vi "Test_Combined_Convert_CameraAngle_to_Flywheel_Velocity.vi"() -> ()   [LabVIEW 2019]
panel:
  in  "angle":dbl
  in  "terminal height":dbl
  out "Test Plot":cluster{dbl[], dbl[]}[](graph)
  out "a2":dbl
  out "d":dbl
  in  "StopValue":dbl=25.0
  in  "StartValue":dbl=-25.0
  in  "h1":dbl=20.56
  in  "h2":dbl=98.25
  in  "a1":dbl
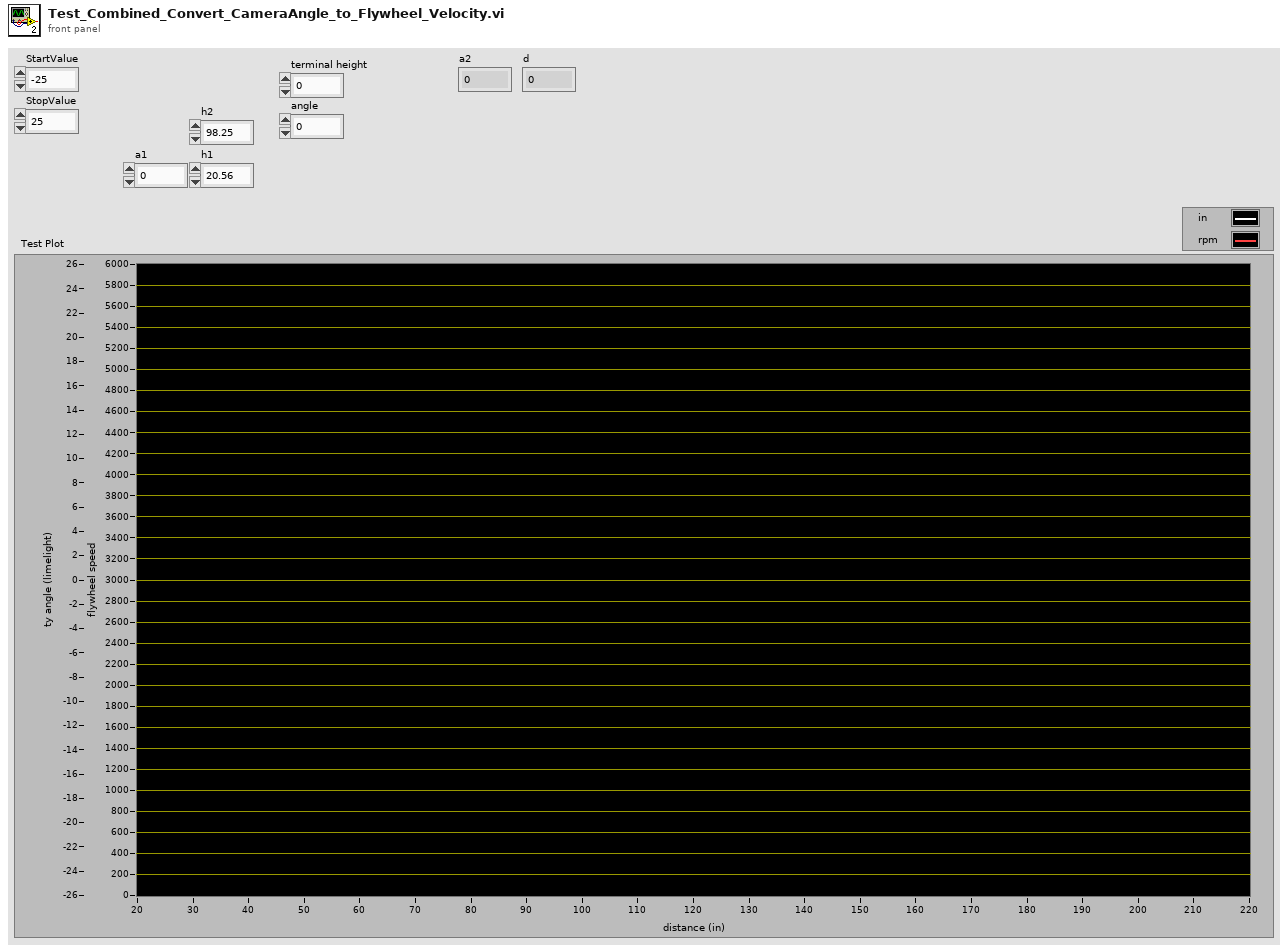
[diagram p1: front panel]
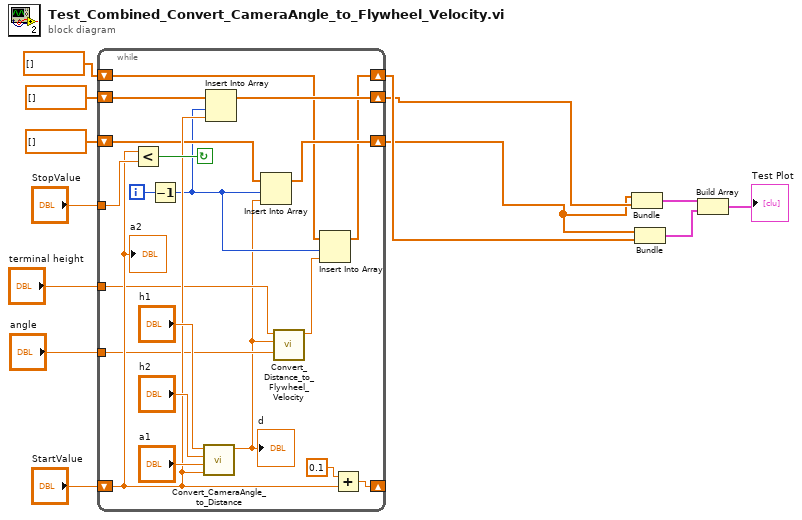
[diagram p0: block diagram]
diagram:
  n1 = while {
    shift-right: [w29] -> _
    shift-left: "StartValue" -> [w25]
    tunnel: "StopValue" -> [w28]
    shift-right: [w22] -> w2
    shift-left: dbl[] [] -> [w24]
    shift-right: [w21] -> w1
    shift-left: dbl[] [] -> [w23]
    shift-right: [w17] -> w3
    shift-left: dbl[] [] -> [w18]
    tunnel: "terminal height" -> [w16]
    tunnel: "angle" -> [w15]
    i -> [w26]
    stop <- w27 continue-if-true
    n2 = Less?(x=w25, y=w28) -> (x < y?=w27:bool)
    n3 = Decrement(x=w26) -> (x-1=w19:i32)
    n4 = call "Convert_CameraAngle_to_Distance.vi"("a2"=w25, "a1"="a1", "h2"="h2", "h1"="h1") -> ("d"=w14:dbl)  [unwired: 7 in]
    "d" <- w14
    n5 = Insert Into Array(array=w24, index=w19, new element=w25) -> (w22:dbl[])
    n6 = Insert Into Array(array=w23, index=w19, new element=w14) -> (w21:dbl[])
    n7 = call "Convert_Distance_to_Flywheel_Velocity.vi"("angle"=w15, "distance"=w14, "terminal height"=w16) -> ("velocity"=w20:dbl)  [unwired: 8 in]
    n8 = Insert Into Array(array=w18, index=w19, new element=w20) -> (w17:dbl[])
    n9 = Add(x=0.1, y=w25) -> (x+y=w29:dbl)
    "a2" <- w25
  }
  n10 = Bundle(w1, w2) -> (w8:cluster{dbl[], dbl[]})  [unwired: 1 in]
  n11 = Bundle(w1, w3) -> (w7:cluster{dbl[], dbl[]})  [unwired: 1 in]
  n12 = Build Array(w8, w7) -> (→"Test Plot":cluster{dbl[], dbl[]}[])
